vi "Host - TX DRAM generation throughput test.vi"() -> ()   [LabVIEW 2019]
uses:
  b31122fc-374d-4bc3-8fea-97b441d8715b.vi
  05a57b60-2ab6-411d-8b9c-a2f9ac5bc040.vi
  56281c02-5be9-4d86-89de-cbc43ae05fbe.vi
  <vilib>/FPGAPlugInAG/PXIe-7902R/niLvFpga_Open_PXIe-7902R.vi
  <vilib>/rvi/interface/common/dynamic/niFpgaDynamicAddResources.vi
  <vilib>/rvi/interface/common/niFpgaWaitOnOcc.vi
  <vilib>/Utility/error.llb/Error Cluster From Error Code.vi
  <vilib>/rvi/errors/niLvFpgaAdjustHostInterfaceError.vi
  <vilib>/FPGAPlugInAG/Dynamic/niLvFpga_Close_Dynamic.vi
  <vilib>/rvi/interface/nirviOpenFPGA/nirviOpenFPGA.xnode
  FPGA Bitfiles/TX_DRAM_generation_throughut_test.lvbitx
  <vilib>/rvi/interface/nirviMethod/nirviMethod.xnode
  <vilib>/rvi/interface/nirviReadWriteControl/nirviReadWriteControl.xnode
  <vilib>/rvi/interface/nirviCloseFPGA/nirviCloseFPGA.xnode
  NiFpgaLv.dll
  <vilib>/rvi/interface/Simulation/niFpgaSimulationCallBeginRW.vi
  <vilib>/FPGAPlugInAG/Dynamic/niLvFpga_ConfigureFifo_Dynamic.vi
  <vilib>/rvi/errors/niLvFpgaMergeErrorWithErrorCode.vi
  <vilib>/FPGAPlugInAG/Dynamic/niLvFpga_WriteFifo_Dynamic.vi
  <vilib>/Analysis/NI_AALBase.lvlib
  <vilib>/FPGAPlugInAG/Dynamic/niLvFpga_ReadFifo_Dynamic.vi
  <vilib>/FPGAPlugInAG/Dynamic/niLvFpga_StartFifo_Dynamic.vi
panel:
  in  "sequence.cont":bool
  in  "debug end":u64=5099
  in  "debug start":u64
  out "gen.pending to read":u32
  out "dram.total req":u32
  out "dram.total rd":u32
  out "dram.total wr":u32
  out "dram.last written addr":u32
  out "dma status":u32
  in  "load time (ms)":u32=2
  in  "repeat":u64=1
  in  "cycles":dbl=10.0
  out "DRAM end addr":i32
  in  "samples":i32=4096
  out "Waveform Graph - Dark":sgl[](graph)
  out "seq.loaded steps":u32
  out "I":fxp<+/-,12,1>[](array[numeric])
  in  "Retrieve":bool
  out "seq.step ctr":u32
  out "seq.state":enum16{"idle", "read step", "execute step"}(ring)
  out "acq samples":u32
  out "missed sample count":u32
  in  "Start sequence":bool
  in  "Wfm addr":u32
  out "size(s)":i32
  in  "Download Button":bool
  out "Status":string
  in  "Stop Button":bool
  in  "RIO Device":tag
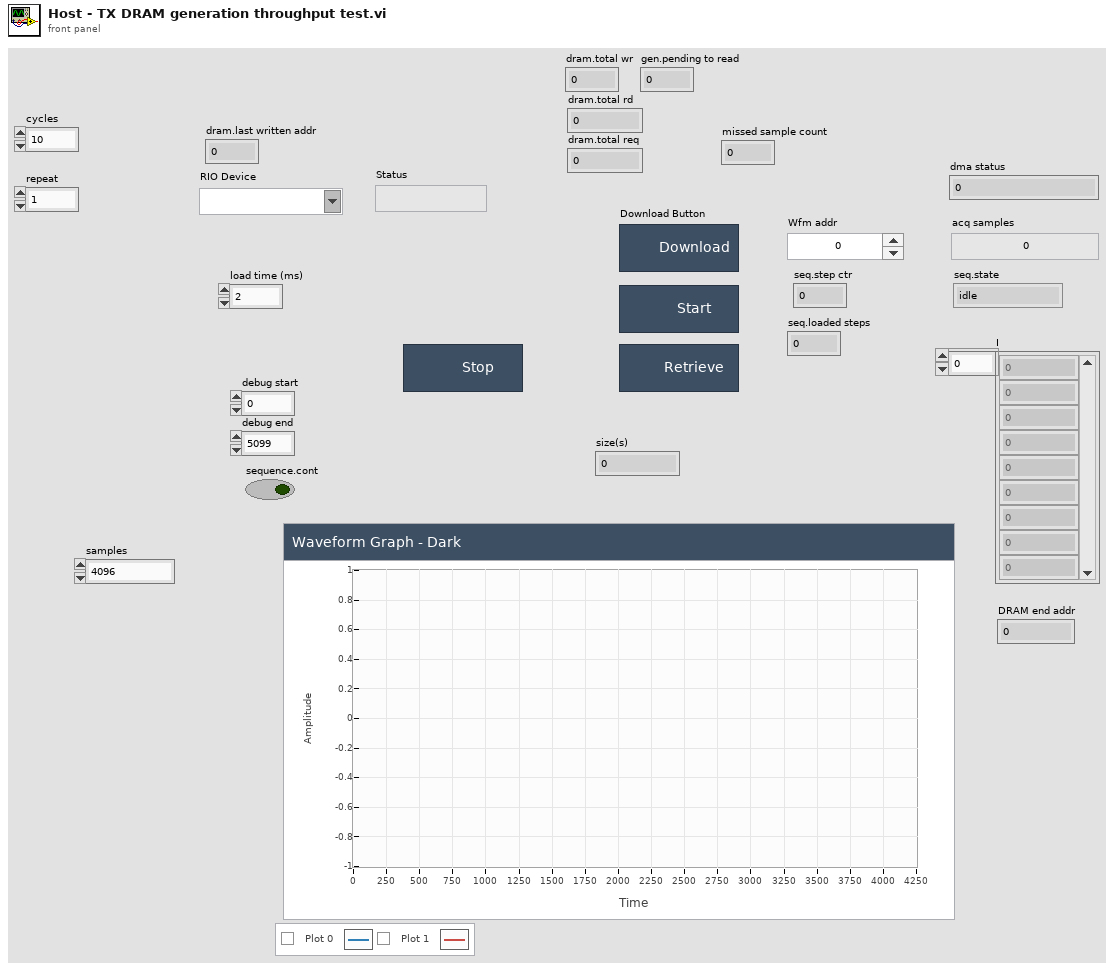
[diagram p1: front panel]
types:
  T1 = cluster{"start addr":u32, "end addr":u32, "repeat":u64}
  T2 = cluster{"total rd":u32, "total wr":u32, "total req":u32}
  T3 = cluster{"fixed-point type":fxp<+/-,12,1>, "fixed-point type":fxp<+/-,12,1>}
  T4 = cluster{"fixed-point type":fxp<+/-,12,1>, "fixed-point type":fxp<+/-,12,1>}[][]
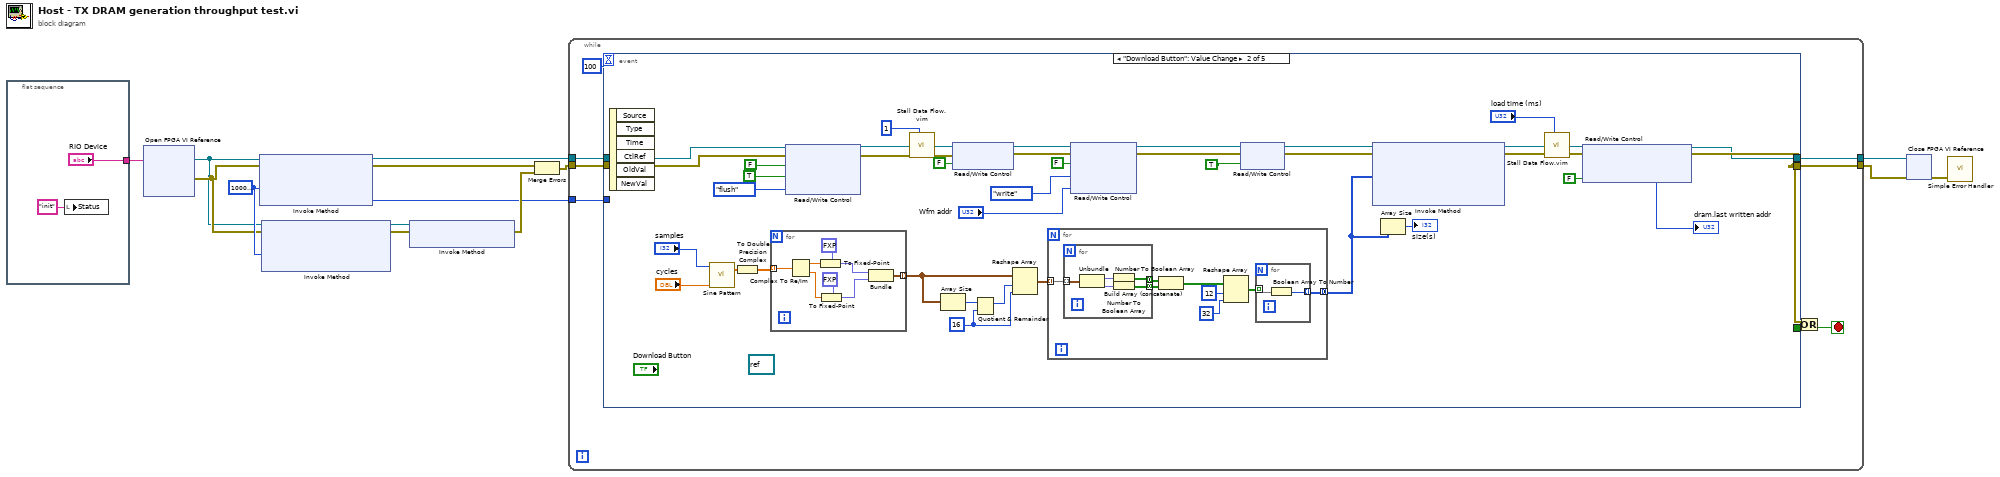
[diagram p0: block diagram]
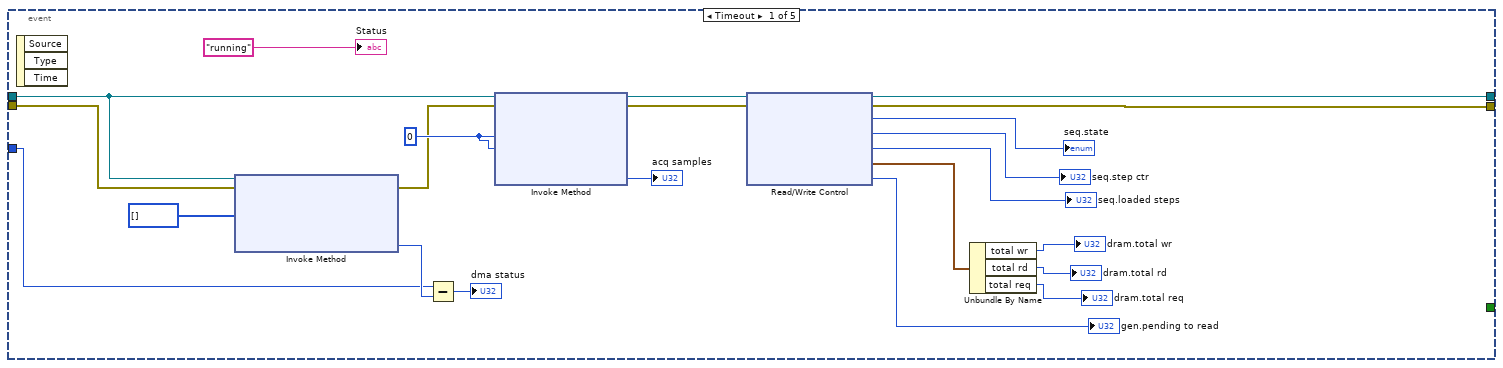
[diagram p2: hidden frame]
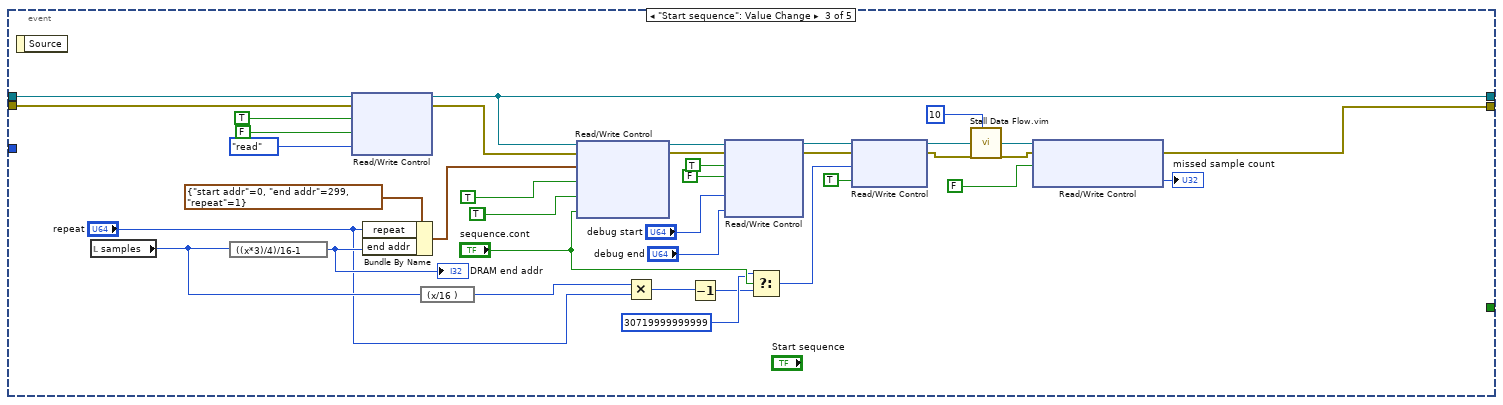
[diagram p3: hidden frame]
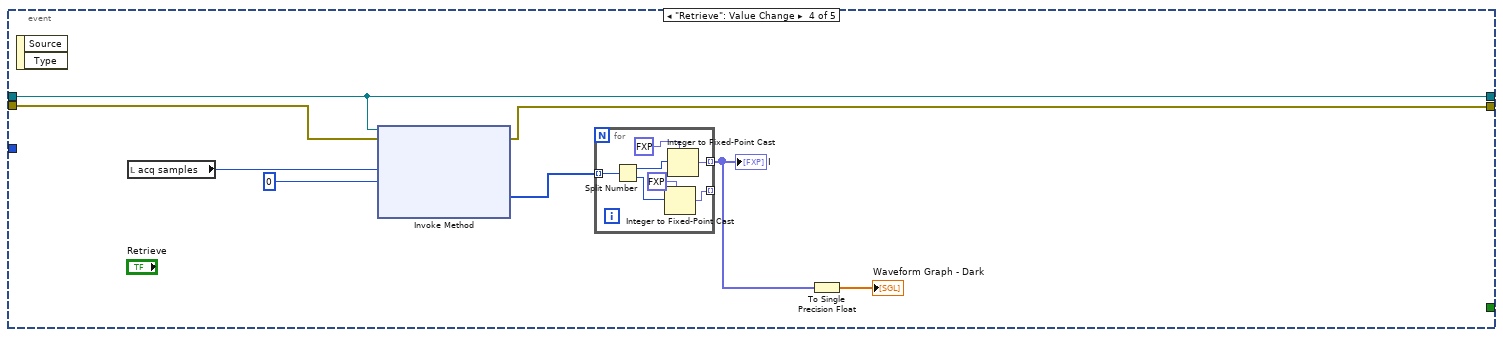
[diagram p4: hidden frame]
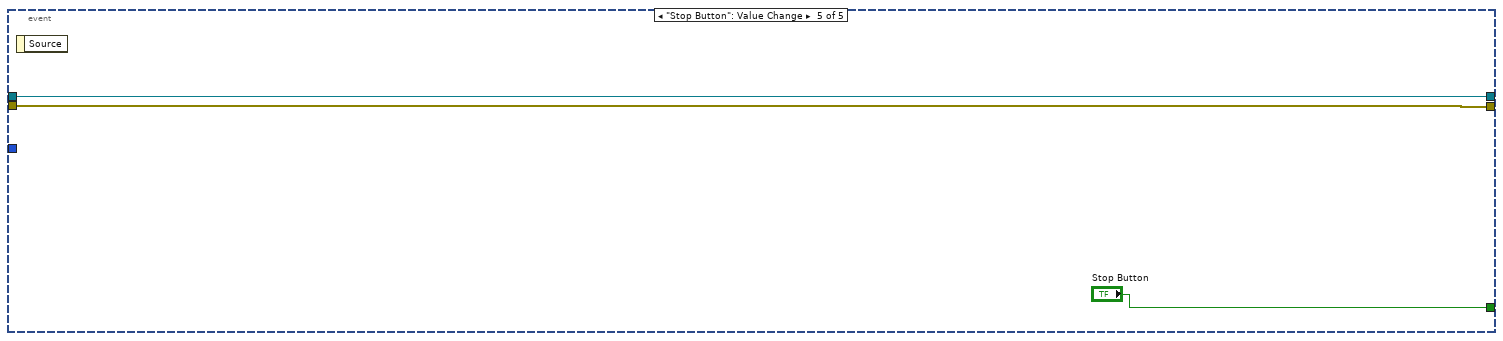
[diagram p5: hidden frame]
diagram:
  w8 = u32 10000000 ("Requested Depth")
  n1 = flat-sequence {
    tunnel: ["RIO Device"] -> w14
    frame #0 {
      n2 = local write "Status"("init" ("Status")) -> ()
    }
  }
  n3 = xnode "Open FPGA VI Reference"("resource name"=w14) -> ("FPGA VI Reference Out"=w6:refnum<k20>, "error out"=w7:errorcluster)  [unwired: 1 in]
  n4 = xnode "Invoke Method"("FPGA VI Reference In"=w6, "error in"=w7, "Requested Depth"=w8) -> ("FPGA VI Reference Out"=w13:refnum<k20>, "error out"=w12:errorcluster, "Actual Depth"=w1:u32)
  n5 = xnode "Invoke Method"("FPGA VI Reference In"=w6, "error in"=w7, "Requested Depth"=w8) -> ("FPGA VI Reference Out"=w5:refnum<k20>, "error out"=w4:errorcluster)  [unwired: 1 out]
  n6 = xnode "Invoke Method"("FPGA VI Reference In"=w5, "error in"=w4) -> ("error out"=w2:errorcluster)  [unwired: 1 out]
  n7 = Merge Errors(w12, w2) -> (w3:errorcluster)
  n8 = while {
    tunnel: w13 -> [w24]
    tunnel: w3 -> [w23]
    tunnel: [w21] -> w11
    tunnel: [w19] -> w10
    tunnel: w1 -> [w17]
    stop <- w20 stop-if-true
    n9 = event shown="[1] \"Download Button\": Value Change" {
      selector: _ -> [_ _ _ _ _]
      dyn-events: _ -> [_ _ _ _ _]
      timeout: 100 -> [_ _ _ _ _]
      tunnel: w24 -> [w36 w73 w131 w151 w160]
      tunnel: w23 -> [w32 w56 w130 w150 w159]
      tunnel: [_ _ _ _ "Stop Button"] -> w22
      tunnel: [w42 w62 w141 w151 w160] -> w21
      tunnel: [w40 w75 w117 w147 w159] -> w19
      tunnel: w17 -> [w33 _ _ _ _]
      event Timeout {
        w44 = u32 0 ("Number of Elements")
        n10 = event-data() -> ()  [unwired: 1 in, 3 out]
        n11 = xnode "Invoke Method"("FPGA VI Reference In"=w36, "error in"=w32, "Data"=u32[] []) -> ("error out"=w31:errorcluster, "Empty Elements Remaining"=w34:u32)  [unwired: 1 in, 1 out]
        n12 = Subtract(x=w33, y=w34) -> (x-y=→"dma status":u32)
        n13 = xnode "Invoke Method"("FPGA VI Reference In"=w36, "error in"=w31, "Number of Elements"=w44, "Timeout (ms)"=w44) -> ("FPGA VI Reference Out"=w45:refnum<k20>, "error out"=w41:errorcluster, "Elements Remaining"=→"acq samples":u32)  [unwired: 1 out]
        n14 = xnode "Read/Write Control"("FPGA VI Reference In"=w45, "error in"=w41) -> ("FPGA VI Reference Out"=w42:refnum<k20>, "error out"=w40:errorcluster, "seq.state"=→"seq.state":enum16{"idle", "read step", "execute step"}, "seq.step ctr"=→"seq.step ctr":u32, "seq.loaded steps"=→"seq.loaded steps":u32, "dram.debug ctr"=w28:T2, "gen.pending to read"=→"gen.pending to read":u32)
        n15 = Unbundle By Name(w28) -> ("total wr"=→"dram.total wr":u32, "total rd"=→"dram.total rd":u32, "total req"=→"dram.total req":u32)
        "Status" <- "running" ("Status")
      }
      event "Download Button": Value Change {
        w52 = 16 ("y")
        (unwired) refnum<k20> refnum ("FPGA VI Reference Out")
        n16 = event-data() -> ()  [unwired: 1 in, 6 out]
        n17 = call <vilib>:"Sine Pattern.vi"("cycles"="cycles", "samples"="samples") -> ("Sinusoidal Pattern"=w84:dbl[])  [unwired: 2 in, 1 out]
        n18 = To Double Precision Complex(1:w84) -> (0:w48:cdb[])
        n19 = for {
          tunnel: w48 -> [w107] mode=indexing
          tunnel: [w105] -> w50 mode=indexing
          n20 = Complex To Re/Im(x + iy=w107) -> (x=w103:dbl, y=w101:dbl)
          n21 = To Fixed-Point(fixed-point type=fxp<+/-,12,1> 0.0, number=w103) -> (fixed-point=w104:fxp<+/-,12,1>)
          n22 = To Fixed-Point(fixed-point type=fxp<+/-,12,1> 0.0, number=w101) -> (fixed-point=w100:fxp<+/-,12,1>)
          n23 = Bundle("fixed-point type"=w104, "fixed-point type"=w100) -> (w105:T3)  [unwired: 1 in]
        }
        n24 = xnode "Read/Write Control"("FPGA VI Reference In"=w73, "error in"=w56, "seq.continous"=FALSE ("sequence.cont"), "dram.reset"=TRUE, "dram mode"=enum16{"flush", "reset", "write", "read"}."flush") -> ("FPGA VI Reference Out"=w70:refnum<k20>, "error out"=w55:errorcluster)
        n25 = call "Stall Data Flow.vim"("value in"=w70, "milliseconds to wait"=u32 1) -> ("value out"=w68:refnum<k20>)  [unwired: 1 out]
        n26 = Array Size(array=w50) -> (size(s)=w49:i32)
        n27 = xnode "Read/Write Control"("FPGA VI Reference In"=w68, "error in"=w55, "dram.reset"=FALSE) -> ("FPGA VI Reference Out"=w69:refnum<k20>, "error out"=w54:errorcluster)
        n28 = Quotient & Remainder(x=w49, y=w52) -> (floor(x/y)=w51:i32)  [unwired: 1 out]
        n29 = Reshape Array(w50, w51, w52) -> (w53:T4)
        n30 = for {
          tunnel: w53 -> [w92] mode=indexing
          tunnel: [w86] -> w47 mode=concatenating
          n31 = for {
            tunnel: w92 -> [w99] mode=indexing
            tunnel: [w97] -> w91 mode=concatenating
            tunnel: [w96] -> w90 mode=concatenating
            n32 = Unbundle(w99) -> ("fixed-point type"=w98:fxp<+/-,12,1>, "fixed-point type"=w95:fxp<+/-,12,1>)
            n33 = Number To Boolean Array(number=w98) -> (Boolean array=w97:bool[])
            n34 = Number To Boolean Array(number=w95) -> (Boolean array=w96:bool[])
          }
          n35 = Build Array (concatenate)(w91, w90) -> (w85:bool[])
          n36 = Reshape Array(w85, 12 ("dimension size"), 32 ("dimension size")) -> (w87:bool[][])
          n37 = for {
            tunnel: w87 -> [w94] mode=indexing
            tunnel: [w93] -> w86 mode=indexing
            n38 = Boolean Array To Number(Boolean array=w94) -> (number=w93:u32)
          }
        }
        n39 = xnode "Read/Write Control"("FPGA VI Reference In"=w69, "error in"=w54, "iq.load"=FALSE, "dram mode"=enum16{"flush", "reset", "write", "read"}."write", "iq.load addr"="Wfm addr") -> ("FPGA VI Reference Out"=w81:refnum<k20>, "error out"=w79:errorcluster)
        n40 = xnode "Read/Write Control"("FPGA VI Reference In"=w81, "error in"=w79, "iq.load"=TRUE ("write/read")) -> ("FPGA VI Reference Out"=w80:refnum<k20>, "error out"=w77:errorcluster)
        n41 = xnode "Invoke Method"("FPGA VI Reference In"=w80, "error in"=w77, "Data"=w47) -> ("FPGA VI Reference Out"=w76:refnum<k20>, "error out"=w75:errorcluster)  [unwired: 1 in, 1 out]
        n42 = Array Size(array=w47) -> (size(s)=→"size(s)":i32)
        n43 = call "Stall Data Flow.vim"("value in"=w76, "milliseconds to wait"="load time (ms)") -> ("value out"=w74:refnum<k20>)  [unwired: 1 out]
        n44 = xnode "Read/Write Control"("FPGA VI Reference In"=w74, "iq.load"=FALSE) -> ("FPGA VI Reference Out"=w62:refnum<k20>, "dram.last written addr"=→"dram.last written addr":u32)  [unwired: 1 in, 1 out]
      }
      event "Start sequence": Value Change {
        (unwired) TRUE ("seq.rst")
        n45 = event-data() -> ()  [unwired: 1 in, 1 out]
        n46 = local read "samples"() -> (w120:i32)
        n47 = expression code="((x*3)/4)/16-1"(w120) -> (w121:i32)
        "DRAM end addr" <- w121
        n48 = xnode "Read/Write Control"("FPGA VI Reference In"=w131, "error in"=w130, "seq.rst"=TRUE, "seq.rst"=FALSE, "dram mode"=enum16{"flush", "reset", "write", "read"}."read") -> ("FPGA VI Reference Out"=w141:refnum<k20>, "error out"=w140:errorcluster)
        n49 = Bundle By Name(cluster=T1 {"start addr"=0, "end addr"=299, "repeat"=1} ("seq.new step"), "repeat"="repeat", "end addr"=w121) -> (w122:T1)
        n50 = expression code="(x/16 )"(w120) -> (w119:i32)
        n51 = xnode "Read/Write Control"("FPGA VI Reference In"=w141, "error in"=w140, "seq.new step"=w122, "seq.add step"=TRUE ("seq.rst"), "seq.add step"=FALSE ("seq.rst"), "seq.continous"="sequence.cont") -> ("FPGA VI Reference Out"=w137:refnum<k20>, "error out"=w136:errorcluster)
        n52 = Multiply(x=w119, y="repeat") -> (x*y=w113:u64)
        n53 = Decrement(x=w113) -> (x-1=w110:u64)
        n54 = xnode "Read/Write Control"("FPGA VI Reference In"=w137, "error in"=w136, "seq.start"=TRUE, "seq.rst"=FALSE ("seq.start"), "debug start"="debug start", "debug end"="debug end") -> ("FPGA VI Reference Out"=w133:refnum<k20>, "error out"=w132:errorcluster)
        n55 = Select(t=u64 30719999999999 ("gen.length"), s="sequence.cont", f=w110) -> (s? t:f=w109:u64)
        n56 = xnode "Read/Write Control"("FPGA VI Reference In"=w133, "error in"=w132, "gen.length"=w109, "gen.start"=TRUE ("seq.start")) -> ("FPGA VI Reference Out"=w128:refnum<k20>, "error out"=w126:errorcluster)
        n57 = call "Stall Data Flow.vim"("value in"=w128, "milliseconds to wait"=u32 10) -> ("value out"=w127:refnum<k20>)  [unwired: 1 out]
        n58 = xnode "Read/Write Control"("FPGA VI Reference In"=w127, "error in"=w126, "gen.start"=FALSE) -> ("error out"=w117:errorcluster, "missed sample count"=→"missed sample count":u32)  [unwired: 1 out]
      }
      event "Retrieve": Value Change {
        n59 = event-data() -> ()  [unwired: 1 in, 2 out]
        n60 = local read "acq samples"() -> (w148:u32)
        n61 = xnode "Invoke Method"("FPGA VI Reference In"=w151, "error in"=w150, "Number of Elements"=w148, "Timeout (ms)"=0) -> ("error out"=w147:errorcluster, "Data"=w146:u32[])  [unwired: 2 out]
        n62 = for {
          tunnel: w146 -> [w158] mode=indexing
          tunnel: [w155] -> w145 mode=indexing
          tunnel: [w152] -> _ mode=indexing
          n63 = Split Number(x=w158) -> (hi(x)=w156:u16, lo(x)=w153:u16)
          n64 = Integer to Fixed-Point Cast(fixed-point type=fxp<+/-,12,1> 0.0, integer=w153) -> (fixed-point=w152:fxp<+/-,12,1>)
          n65 = Integer to Fixed-Point Cast(fixed-point type=fxp<+/-,12,1> 0.0, integer=w156) -> (fixed-point=w155:fxp<+/-,12,1>)
        }
        "I" <- w145
        n66 = To Single Precision Float(number=w145) -> (single precision float=→"Waveform Graph - Dark":sgl[])
      }
      event "Stop Button": Value Change {
        n67 = event-data() -> ()  [unwired: 1 in, 1 out]
      }
    }
    n68 = Or(x=w19, y=w22) -> (x .or. y?=w20:bool)
  }
  n69 = xnode "Close FPGA VI Reference"("FPGA VI Reference In"=w11, "error in"=w10) -> ("error out"=w9:errorcluster)
  n70 = call <vilib>:"Simple Error Handler.vi"("error in (no error)"=w9) -> ()  [unwired: 4 in, 5 out]
